vi "Experiment Diagram.vi"   [LabVIEW 2016]
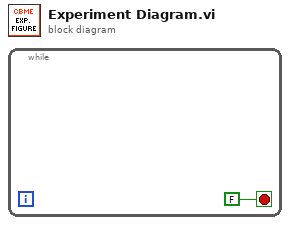
[diagram p0: block diagram]
diagram:
  n1 = while {
    stop <- FALSE stop-if-true
  }
